vi "模拟发送.vi"() -> ()   [LabVIEW 2013]
panel:
  out "发送成功":bool
  in  "清空":bool
  in  "全选":bool
  in  "DO模块故障":enum16{"无", "一级", "二级", "三级"}(ring) caption="电压检测模块故障"
  in  "DI模块故障":enum16{"无", "一级", "二级", "三级"}(ring) caption="电压检测模块故障"
  in  "软件故障":enum16{"无", "一级", "二级", "三级"}(ring) caption="电压检测模块故障"
  in  "放电均衡模块故障":enum16{"无", "一级", "二级", "三级"}(ring) caption="电压检测模块故障"
  in  "充电均衡模块故障":enum16{"无", "一级", "二级", "三级"}(ring) caption="电压检测模块故障"
  in  "CAN1通讯模块故障":enum16{"无", "一级", "二级", "三级"}(ring) caption="电压检测模块故障"
  in  "CAN0通讯模块故障":enum16{"无", "一级", "二级", "三级"}(ring) caption="电压检测模块故障"
  in  "CAN4通讯模块故障":enum16{"无", "一级", "二级", "三级"}(ring) caption="电压检测模块故障"
  in  "CPU故障":enum16{"无", "一级", "二级", "三级"}(ring) caption="电压检测模块故障"
  in  "CPU内部FLASH存储器故障":enum16{"无", "一级", "二级", "三级"}(ring) caption="电压检测模块故障"
  in  "45db041存储器故障":enum16{"无", "一级", "二级", "三级"}(ring) caption="电压检测模块故障"
  in  "EE存储器故障":enum16{"无", "一级", "二级", "三级"}(ring) caption="电压检测模块故障"
  in  "CPU内部EE故障":enum16{"无", "一级", "二级", "三级"}(ring) caption="电压检测模块故障"
  in  "系统外扩时钟模块故障":enum16{"无", "一级", "二级", "三级"}(ring) caption="电压检测模块故障"
  in  "外总压检测模块故障":enum16{"无", "一级", "二级", "三级"}(ring) caption="电压检测模块故障"
  in  "内总压检测模块故障":enum16{"无", "一级", "二级", "三级"}(ring) caption="电压检测模块故障"
  in  "绝缘检测模块故障":enum16{"无", "一级", "二级", "三级"}(ring) caption="电压检测模块故障"
  in  "电流检测模块故障":enum16{"无", "一级", "二级", "三级"}(ring) caption="电压检测模块故障"
  in  "温度检测模块故障":enum16{"无", "一级", "二级", "三级"}(ring) caption="电压检测模块故障"
  in  "电压检测模块故障":enum16{"无", "一级", "二级", "三级"}(ring)
  in  "默认":bool
  in  "从板板号":T1(ring)
  in  "SOH":i32
  in  "SOC":i32
  in  "放电总安时":dbl
  in  "充电总安时":dbl
  in  "平均电流 2":dbl caption="平均电流"
  in  "外总压 2":dbl caption="外总压"
  in  "总电流 2":dbl caption="总电流"
  in  "总电压 2":dbl caption="总电压"
  out "硬件故障":string
  in  "位置":i32
  in  "最小温度":dbl
  in  "位置":i32
  in  "最大温度":dbl
  in  "位置":i32
  in  "最小电压":dbl
  in  "位置":i32
  in  "最大电压":dbl
  in  "平均电流":dbl
  in  "外总压":dbl
  in  "总电流":dbl
  in  "总电压":dbl
  out "LIFE":i32
  in  "开始":bool
  in  "停止":bool
  # "从板数据"
  # "高压数据"
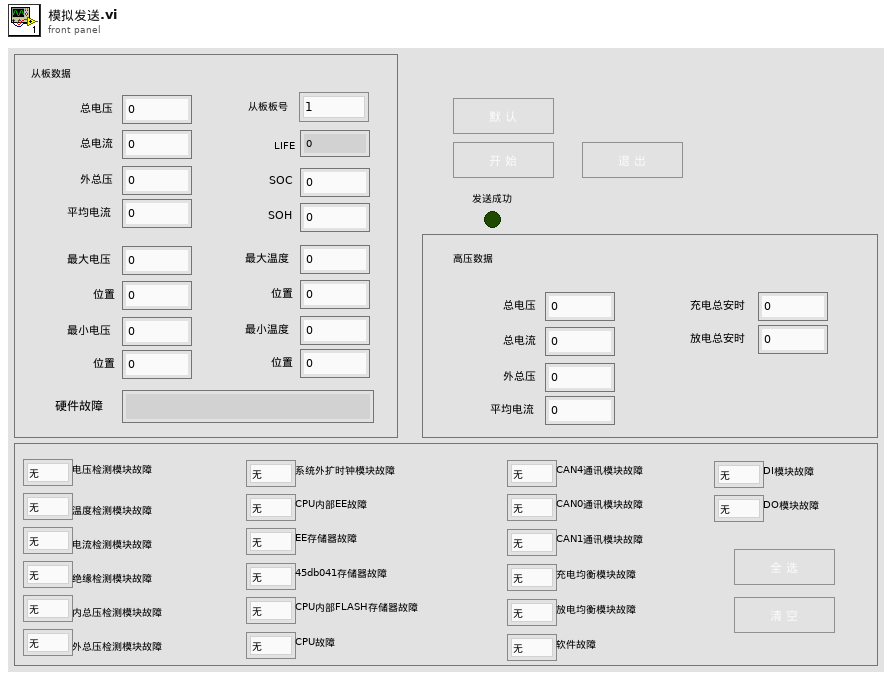
[diagram p1: front panel]
types:
  T1 = enum16{"1", "2", "3", "4", "5", "6", "7", "8", "9", "10", "11", "12", "13", "14", "15", "16", "17", "18", "19", "20", "21", "22", "23", "24", "25", "26", "27", "28", "29", "30"}
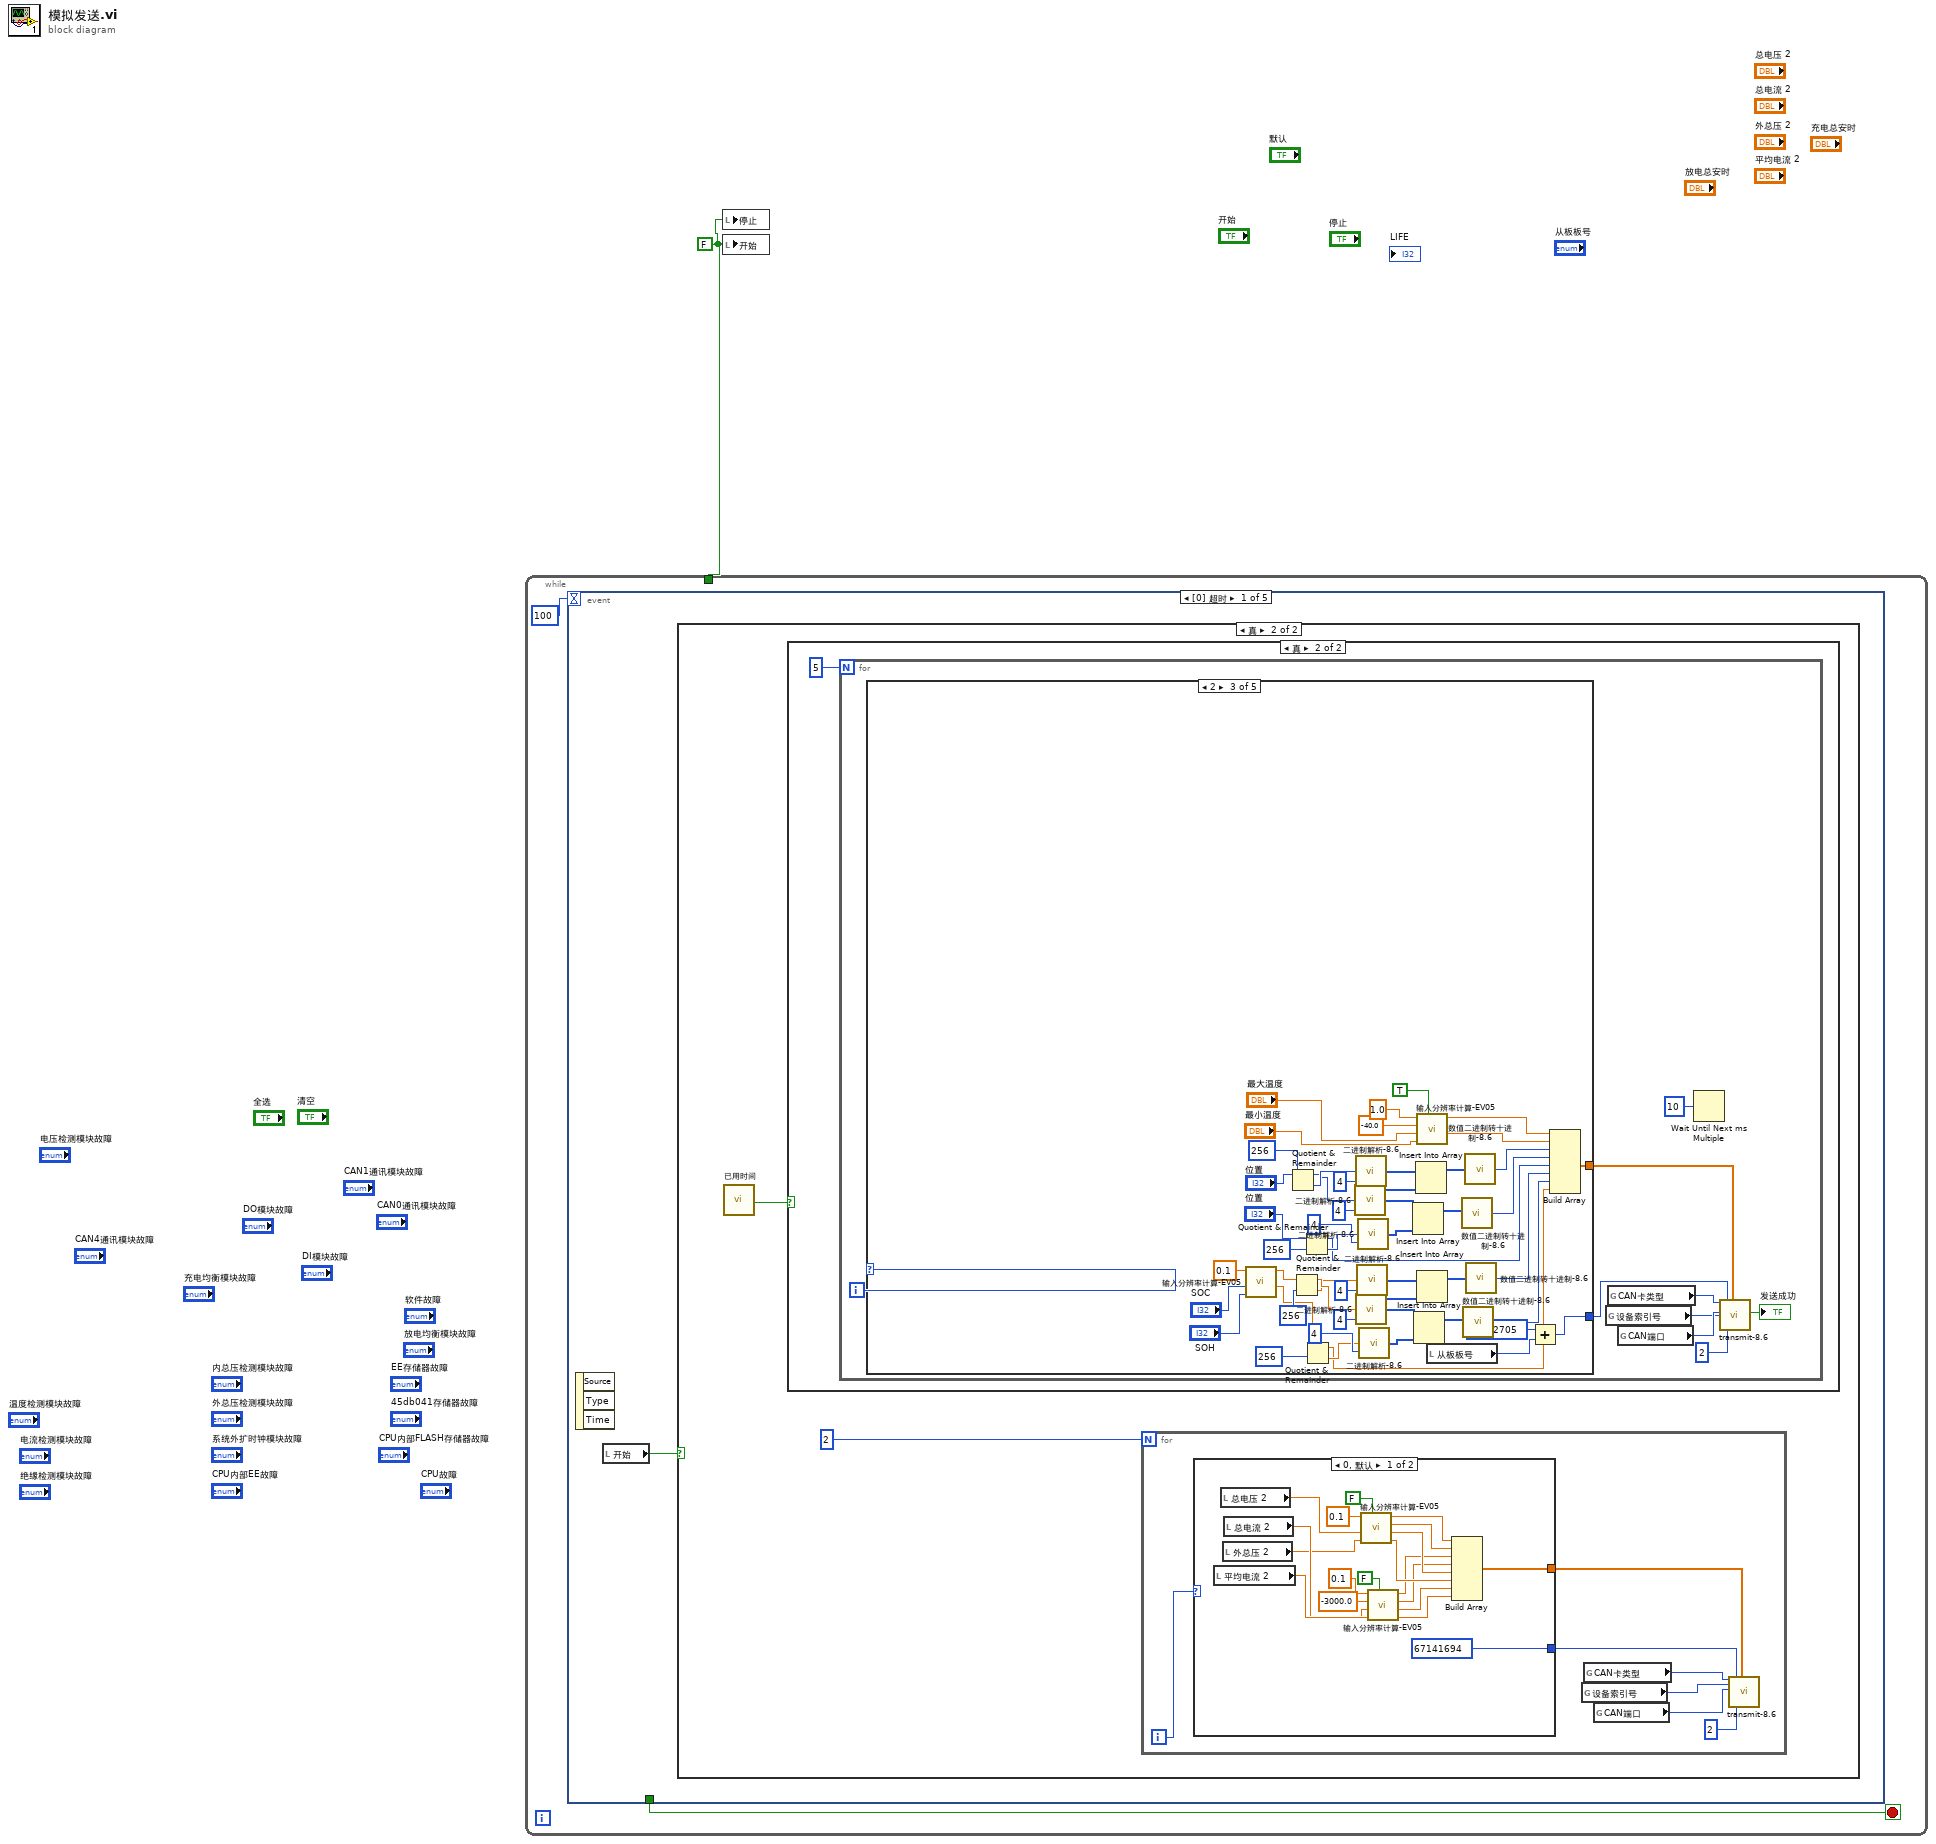
[diagram p0: block diagram]
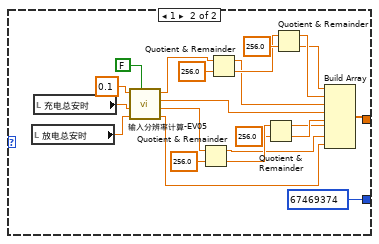
[diagram p3: hidden frame]
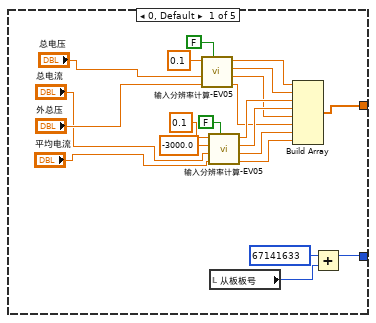
[diagram p5: hidden frame]
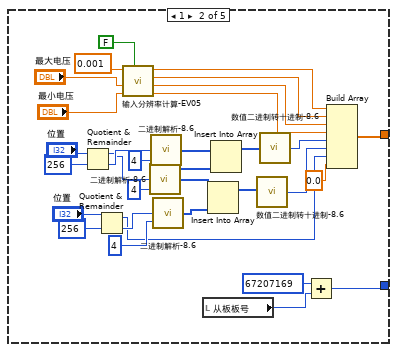
[diagram p6: hidden frame]
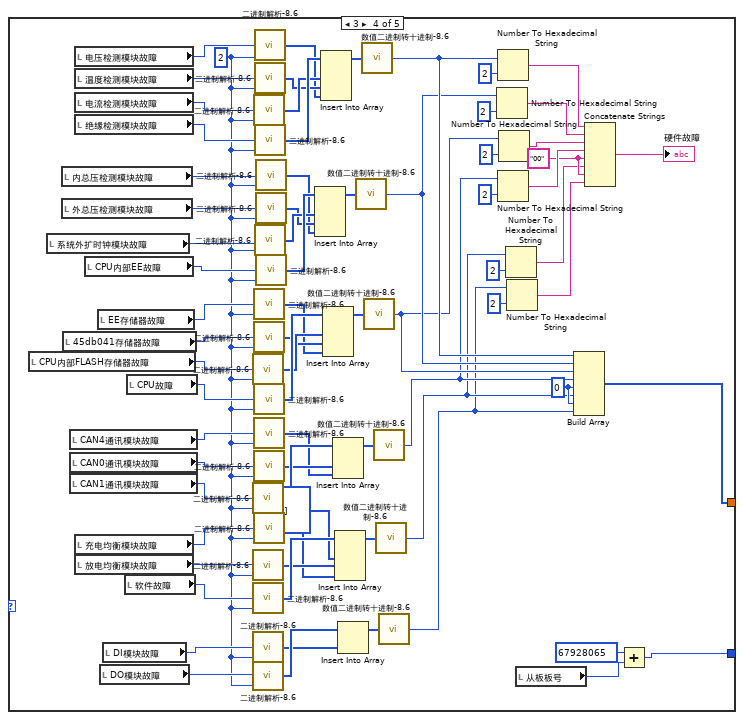
[diagram p7: hidden frame]
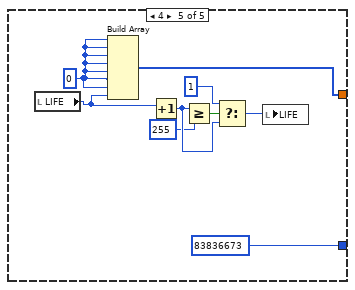
[diagram p8: hidden frame]
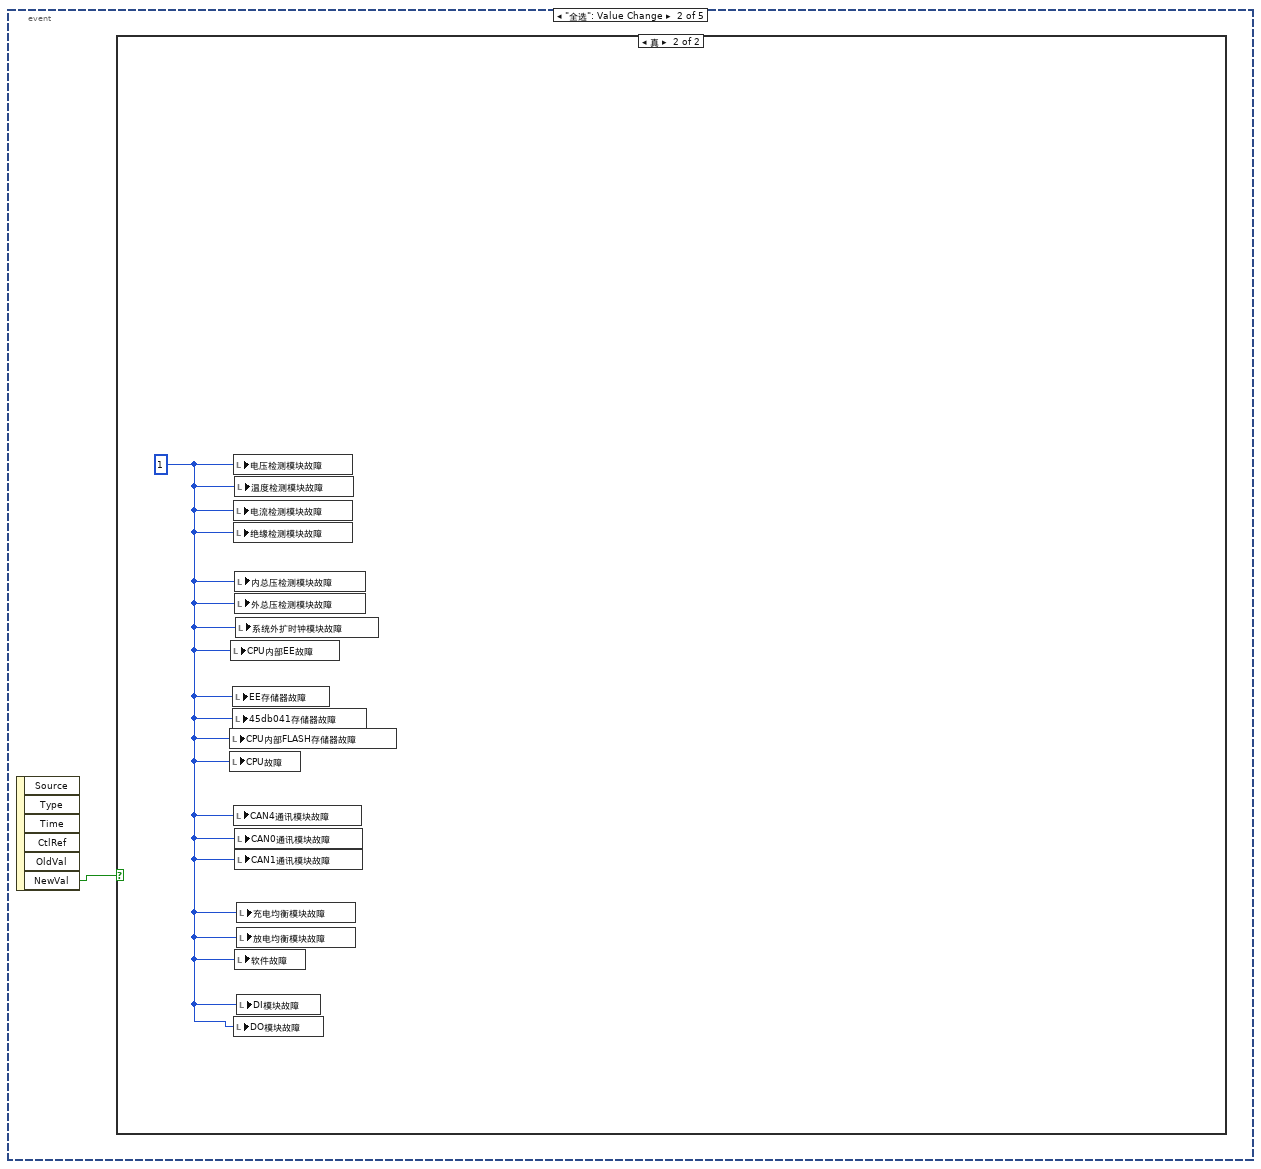
[diagram p9: hidden frame]
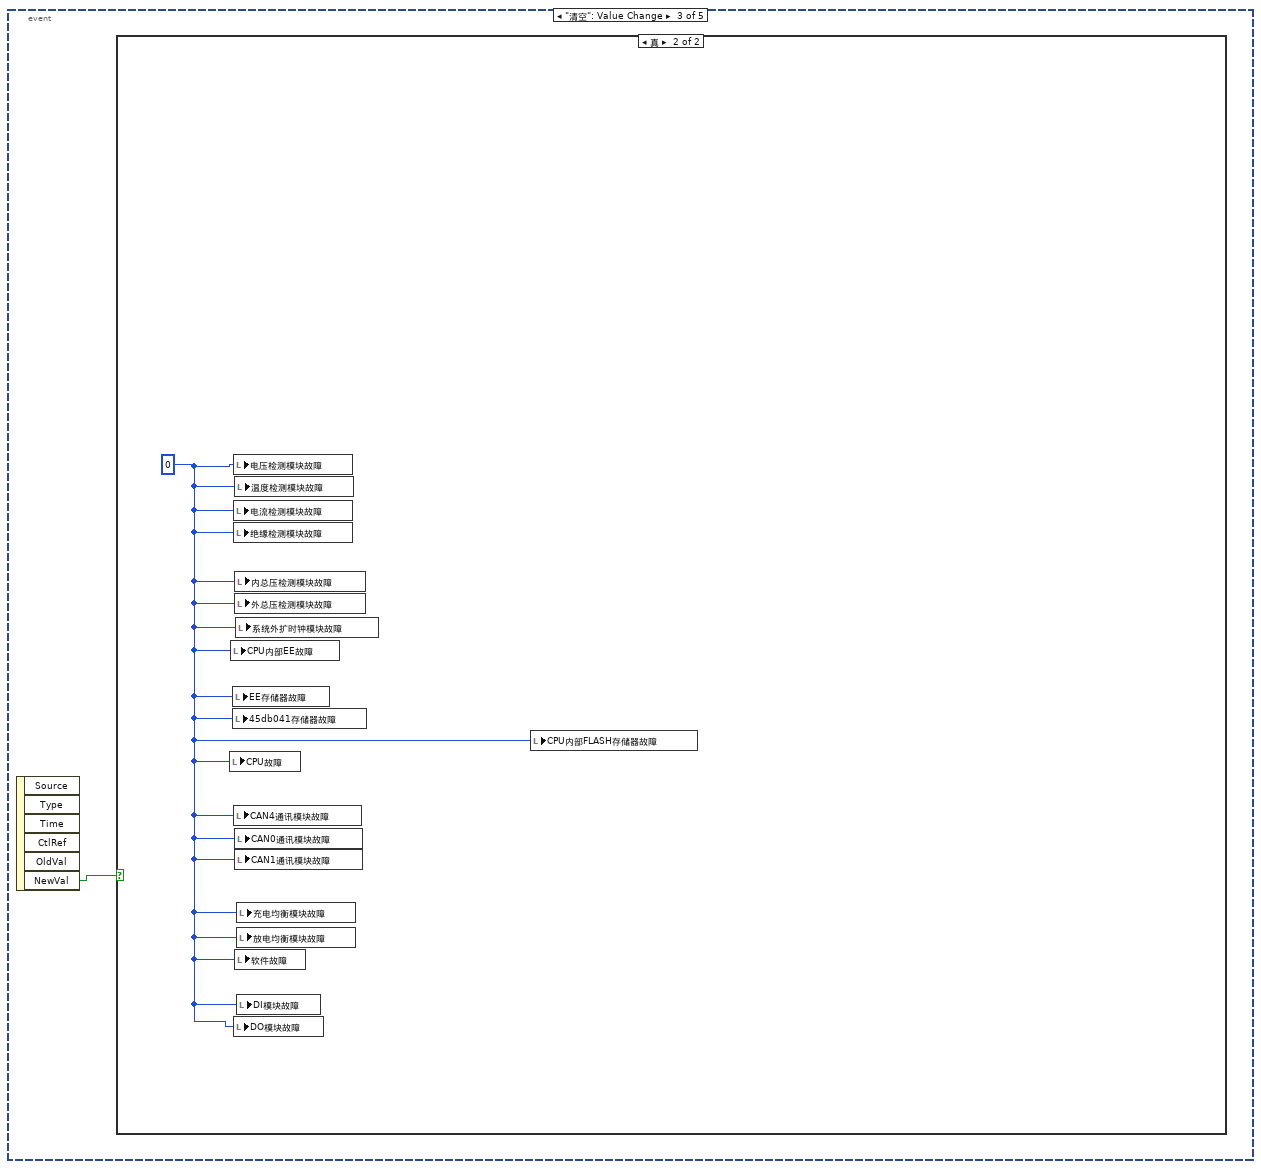
[diagram p11: hidden frame]
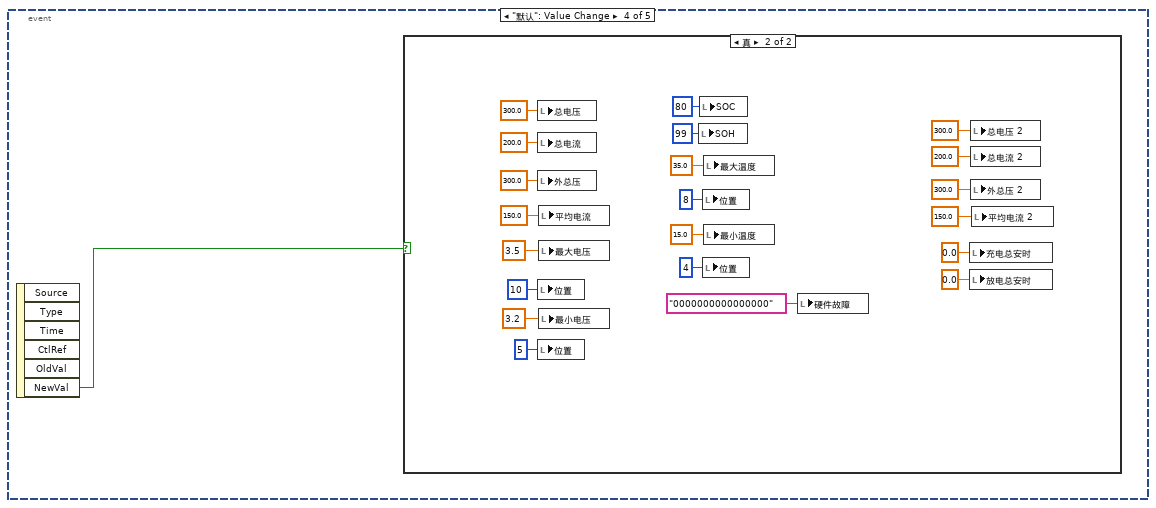
[diagram p13: hidden frame]
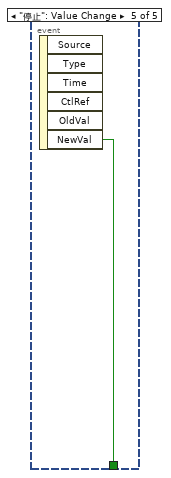
[diagram p15: hidden frame]
diagram:
  w1 = FALSE ("开始")
  n1 = while {
    tunnel: w1 -> [_]
    stop <- w2 stop-if-true
    n2 = event shown="[0] 超时" {
      selector: _ -> [_ _ _ _ _]
      dyn-events: _ -> [_ _ _ _ _]
      timeout: 100 -> [_ _ _ _ _]
      tunnel: [_ _ _ _ w278] -> w2
      event Timeout {
        n3 = event-data() -> ()  [unwired: 1 in, 3 out]
        n4 = local read "开始"() -> (w4:bool)
        n5 = case shown="真" w4 {
          frame False {
          }
          frame True {
            n6 = call "已用时间"() -> ("Time has Elapsed"=w6:bool)  [unwired: 12 in, 7 out]
            n7 = case shown="真" w6 {
              frame False {
              }
              frame True {
                n8 = for {
                  N: 5 -> [_]
                  i -> [w64]
                  n9 = case shown="2" w64 {
                    tunnel: [w69 w113 w169 w190 w244] -> w58
                    tunnel: [w84 w86 w123 w240 83836673] -> w59
                    frame 0, Default {
                      n10 = call "输入分辨率计算-EV05.vi"("1字节?"=FALSE, "数值 2"="外总压", "数值"="总电压", "分辨率"=0.1) -> ("低字节 2"=w72:dbl, "高字节 2"=w73:dbl, "低字节"=w76:dbl, "高字节1"=w77:dbl)  [unwired: 4 in]
                      n11 = call "输入分辨率计算-EV05.vi"("1字节?"=FALSE, "数值 2"="平均电流", "数值"="总电流", "偏移量"=-3000.0, "分辨率"=0.1) -> ("低字节 2"=w70:dbl, "高字节 2"=w71:dbl, "低字节"=w74:dbl, "高字节1"=w75:dbl)  [unwired: 3 in]
                      n12 = local read "从板板号"() -> (w83:T1)
                      n13 = Build Array(w77, w76, w75, w74, w73, w72, w71, w70) -> (w69:dbl[])
                      n14 = Add(x=67141633, y=w83) -> (x+y=w84:i32)
                    }
                    frame 1 {
                      n15 = Quotient & Remainder(x="位置", y=256) -> (x-y*floor(x/y)=w105:i32, floor(x/y)=w108:i32)
                      n16 = Quotient & Remainder(x="位置", y=256) -> (x-y*floor(x/y)=w90:i32, floor(x/y)=w96:i32)
                      n17 = call "输入分辨率计算-EV05.vi"("1字节?"=FALSE, "数值 2"="最小电压", "数值"="最大电压", "分辨率"=0.001) -> ("低字节 2"=w97:dbl, "高字节 2"=w98:dbl, "低字节"=w99:dbl, "高字节1"=w100:dbl)  [unwired: 4 in]
                      n18 = call "二进制解析-8.6.vi"("索引"=4, "数值"=w105) -> ("低位子数组"=w93:i32[], "高位子数组"=w103:i32[])  [unwired: 1 in, 1 out]
                      n19 = call "二进制解析-8.6.vi"("索引"=4, "数值"=w108) -> ("低位子数组"=w104:i32[])  [unwired: 1 in, 2 out]
                      n20 = call "二进制解析-8.6.vi"("索引"=4, "数值"=w96) -> ("低位子数组"=w94:i32[])  [unwired: 1 in, 2 out]
                      n21 = local read "从板板号"() -> (w87:T1)
                      n22 = Insert Into Array(array=w93, new element=w94) -> (w92:i32[])  [unwired: 1 in]
                      n23 = Insert Into Array(array=w104, new element=w103) -> (w102:i32[])  [unwired: 1 in]
                      n24 = call "数值二进制转十进制-8.6.vi"("子数组"=w92) -> ("十进制数值"=w91:i32)  [unwired: 4 in]
                      n25 = call "数值二进制转十进制-8.6.vi"("子数组"=w102) -> ("十进制数值"=w101:i32)  [unwired: 4 in]
                      n26 = Add(x=67207169, y=w87) -> (x+y=w86:i32)
                      n27 = Build Array(w100, w99, w98, w97, w101, w91, w90, 0.0 ("元素")) -> (w113:dbl[])
                    }
                    frame 2 {
                      n28 = call "输入分辨率计算-EV05.vi"("数值 2"="SOH", "数值"="SOC", "分辨率"=0.1) -> ("高字节 2"=w119:dbl, "高字节1"=w120:dbl)  [unwired: 5 in, 2 out]
                      n29 = Quotient & Remainder(x="位置", y=256) -> (x-y*floor(x/y)=w158:i32, floor(x/y)=w161:i32)
                      n30 = Quotient & Remainder(x=w120, y=256) -> (x-y*floor(x/y)=w134:dbl, floor(x/y)=w131:dbl)
                      n31 = Quotient & Remainder(x="位置", y=256) -> (x-y*floor(x/y)=w143:i32, floor(x/y)=w154:i32)
                      n32 = Quotient & Remainder(x=w119, y=256) -> (x-y*floor(x/y)=w128:dbl, floor(x/y)=w138:dbl)
                      n33 = call "二进制解析-8.6.vi"("索引"=4, "数值"=w158) -> ("低位子数组"=w151:i32[], "高位子数组"=w156:i32[])  [unwired: 1 in, 1 out]
                      n34 = call "二进制解析-8.6.vi"("索引"=4, "数值"=w161) -> ("低位子数组"=w157:i32[])  [unwired: 1 in, 2 out]
                      n35 = call "二进制解析-8.6.vi"("索引"=4, "数值"=w134) -> ("低位子数组"=w141:i32[], "高位子数组"=w136:i32[])  [unwired: 1 in, 1 out]
                      n36 = call "二进制解析-8.6.vi"("索引"=4, "数值"=w131) -> ("低位子数组"=w135:i32[])  [unwired: 1 in, 2 out]
                      n37 = call "二进制解析-8.6.vi"("索引"=4, "数值"=w154) -> ("低位子数组"=w152:i32[])  [unwired: 1 in, 2 out]
                      n38 = call "二进制解析-8.6.vi"("索引"=4, "数值"=w138) -> ("低位子数组"=w140:i32[])  [unwired: 1 in, 2 out]
                      n39 = Insert Into Array(array=w151, new element=w152) -> (w150:i32[])  [unwired: 1 in]
                      n40 = Insert Into Array(array=w141, new element=w140) -> (w142:i32[])  [unwired: 1 in]
                      n41 = Insert Into Array(array=w157, new element=w156) -> (w155:i32[])  [unwired: 1 in]
                      n42 = call "输入分辨率计算-EV05.vi"("1字节?"=TRUE, "数值 2"="最小温度", "数值"="最大温度", "偏移量"=-40.0, "分辨率"=1.0) -> ("高字节 2"=w162:dbl, "高字节1"=w163:dbl)  [unwired: 3 in, 2 out]
                      n43 = Insert Into Array(array=w135, new element=w136) -> (w137:i32[])  [unwired: 1 in]
                      n44 = local read "从板板号"() -> (w124:T1)
                      n45 = call "数值二进制转十进制-8.6.vi"("子数组"=w150) -> ("十进制数值"=w144:i32)  [unwired: 4 in]
                      n46 = call "数值二进制转十进制-8.6.vi"("子数组"=w142) -> ("十进制数值"=w127:i32)  [unwired: 4 in]
                      n47 = call "数值二进制转十进制-8.6.vi"("子数组"=w155) -> ("十进制数值"=w145:i32)  [unwired: 4 in]
                      n48 = call "数值二进制转十进制-8.6.vi"("子数组"=w137) -> ("十进制数值"=w126:i32)  [unwired: 4 in]
                      n49 = Add(x=67272705, y=w124) -> (x+y=w123:i32)
                      n50 = Build Array(w163, w162, w145, w144, w143, w126, w127, w128) -> (w169:dbl[])
                    }
                    frame 3 {
                      w172 = "00" ("字符串")
                      w189 = 0 ("元素")
                      w219 = 2
                      n51 = local read "CPU内部FLASH存储器故障"() -> (w229:enum16{"无", "一级", "二级", "三级"})
                      n52 = local read "系统外扩时钟模块故障"() -> (w233:enum16{"无", "一级", "二级", "三级"})
                      n53 = local read "内总压检测模块故障"() -> (w235:enum16{"无", "一级", "二级", "三级"})
                      n54 = local read "外总压检测模块故障"() -> (w234:enum16{"无", "一级", "二级", "三级"})
                      n55 = local read "45db041存储器故障"() -> (w230:enum16{"无", "一级", "二级", "三级"})
                      n56 = local read "CAN4通讯模块故障"() -> (w227:enum16{"无", "一级", "二级", "三级"})
                      n57 = local read "CAN0通讯模块故障"() -> (w226:enum16{"无", "一级", "二级", "三级"})
                      n58 = local read "CAN1通讯模块故障"() -> (w225:enum16{"无", "一级", "二级", "三级"})
                      n59 = local read "电压检测模块故障"() -> (w239:enum16{"无", "一级", "二级", "三级"})
                      n60 = local read "温度检测模块故障"() -> (w238:enum16{"无", "一级", "二级", "三级"})
                      n61 = local read "电流检测模块故障"() -> (w237:enum16{"无", "一级", "二级", "三级"})
                      n62 = local read "绝缘检测模块故障"() -> (w236:enum16{"无", "一级", "二级", "三级"})
                      n63 = local read "充电均衡模块故障"() -> (w224:enum16{"无", "一级", "二级", "三级"})
                      n64 = local read "放电均衡模块故障"() -> (w223:enum16{"无", "一级", "二级", "三级"})
                      n65 = local read "CPU内部EE故障"() -> (w232:enum16{"无", "一级", "二级", "三级"})
                      n66 = local read "EE存储器故障"() -> (w231:enum16{"无", "一级", "二级", "三级"})
                      n67 = local read "DO模块故障"() -> (w220:enum16{"无", "一级", "二级", "三级"})
                      n68 = local read "DI模块故障"() -> (w221:enum16{"无", "一级", "二级", "三级"})
                      n69 = local read "软件故障"() -> (w222:enum16{"无", "一级", "二级", "三级"})
                      n70 = local read "CPU故障"() -> (w228:enum16{"无", "一级", "二级", "三级"})
                      n71 = call "二进制解析-8.6.vi"("索引"=w219, "数值"=w229) -> ("低位子数组"=w202:i32[])  [unwired: 1 in, 2 out]
                      n72 = call "二进制解析-8.6.vi"("索引"=w219, "数值"=w225) -> ("低位子数组"=w198:i32[])  [unwired: 1 in, 2 out]
                      n73 = call "二进制解析-8.6.vi"("索引"=w219, "数值"=w223) -> ("低位子数组"=w193:i32[])  [unwired: 1 in, 2 out]
                      n74 = call "二进制解析-8.6.vi"("索引"=w219, "数值"=w222) -> ("低位子数组"=w194:i32[])  [unwired: 1 in, 2 out]
                      n75 = call "二进制解析-8.6.vi"("索引"=w219, "数值"=w221) -> ("低位子数组"=w186:i32[])  [unwired: 1 in, 2 out]
                      n76 = call "二进制解析-8.6.vi"("索引"=w219, "数值"=w220) -> ("低位子数组"=w187:i32[])  [unwired: 1 in, 2 out]
                      n77 = call "二进制解析-8.6.vi"("索引"=w219, "数值"=w237) -> ("低位子数组"=w211:i32[])  [unwired: 1 in, 2 out]
                      n78 = call "二进制解析-8.6.vi"("索引"=w219, "数值"=w231) -> ("低位子数组"=w200:i32[])  [unwired: 1 in, 2 out]
                      n79 = call "二进制解析-8.6.vi"("索引"=w219, "数值"=w230) -> ("低位子数组"=w201:i32[])  [unwired: 1 in, 2 out]
                      n80 = call "二进制解析-8.6.vi"("索引"=w219, "数值"=w228) -> ("低位子数组"=w203:i32[])  [unwired: 1 in, 2 out]
                      n81 = call "二进制解析-8.6.vi"("索引"=w219, "数值"=w227) -> ("低位子数组"=w196:i32[])  [unwired: 1 in, 2 out]
                      n82 = call "二进制解析-8.6.vi"("索引"=w219, "数值"=w226) -> ("低位子数组"=w197:i32[])  [unwired: 1 in, 2 out]
                      n83 = call "二进制解析-8.6.vi"("索引"=w219, "数值"=w224) -> ("低位子数组"=w192:i32[])  [unwired: 1 in, 2 out]
                      n84 = call "二进制解析-8.6.vi"("索引"=w219, "数值"=w239) -> ("低位子数组"=w209:i32[])  [unwired: 1 in, 2 out]
                      n85 = call "二进制解析-8.6.vi"("索引"=w219, "数值"=w238) -> ("低位子数组"=w210:i32[])  [unwired: 1 in, 2 out]
                      n86 = call "二进制解析-8.6.vi"("索引"=w219, "数值"=w236) -> ("低位子数组"=w212:i32[])  [unwired: 1 in, 2 out]
                      n87 = call "二进制解析-8.6.vi"("索引"=w219, "数值"=w233) -> ("低位子数组"=w207:i32[])  [unwired: 1 in, 2 out]
                      n88 = call "二进制解析-8.6.vi"("索引"=w219, "数值"=w235) -> ("低位子数组"=w205:i32[])  [unwired: 1 in, 2 out]
                      n89 = call "二进制解析-8.6.vi"("索引"=w219, "数值"=w234) -> ("低位子数组"=w206:i32[])  [unwired: 1 in, 2 out]
                      n90 = call "二进制解析-8.6.vi"("索引"=w219, "数值"=w232) -> ("低位子数组"=w208:i32[])  [unwired: 1 in, 2 out]
                      n91 = Insert Into Array(array=w208, new element #1=w207, new element #2=w206, new element #3=w205) -> (w213:i32[])  [unwired: 1 in]
                      n92 = Insert Into Array(array=w212, new element #1=w211, new element #2=w210, new element #3=w209) -> (w218:i32[])  [unwired: 1 in]
                      n93 = Insert Into Array(array=w203, new element #1=w202, new element #2=w201, new element #3=w200) -> (w204:i32[])  [unwired: 1 in]
                      n94 = Insert Into Array(array=w198, new element #1=w197, new element #2=w196) -> (w199:i32[])  [unwired: 1 in]
                      n95 = Insert Into Array(array=w194, new element #1=i32[] [0, 0], new element #2=w193, new element #3=w192) -> (w195:i32[])  [unwired: 1 in]
                      n96 = Insert Into Array(array=w187, new element=w186) -> (w188:i32[])  [unwired: 1 in]
                      n97 = call "数值二进制转十进制-8.6.vi"("子数组"=w213) -> ("十进制数值"=w180:i32)  [unwired: 4 in]
                      n98 = call "数值二进制转十进制-8.6.vi"("子数组"=w218) -> ("十进制数值"=w214:i32)  [unwired: 4 in]
                      n99 = call "数值二进制转十进制-8.6.vi"("子数组"=w204) -> ("十进制数值"=w179:i32)  [unwired: 4 in]
                      n100 = call "数值二进制转十进制-8.6.vi"("子数组"=w199) -> ("十进制数值"=w178:i32)  [unwired: 4 in]
                      n101 = call "数值二进制转十进制-8.6.vi"("子数组"=w195) -> ("十进制数值"=w177:i32)  [unwired: 4 in]
                      n102 = call "数值二进制转十进制-8.6.vi"("子数组"=w188) -> ("十进制数值"=w176:i32)  [unwired: 4 in]
                      n103 = Number To Hexadecimal String(1:i16 2 ("宽度(-)"), 2:w180) -> (0:w175:string)
                      n104 = Number To Hexadecimal String(1:i16 2 ("宽度(-)"), 2:w214) -> (0:w216:string)
                      n105 = Number To Hexadecimal String(1:i16 2 ("宽度(-)"), 2:w178) -> (0:w173:string)
                      n106 = Number To Hexadecimal String(1:i16 2 ("宽度(-)"), 2:w179) -> (0:w174:string)
                      n107 = Number To Hexadecimal String(1:i16 2 ("宽度(-)"), 2:w177) -> (0:w171:string)
                      n108 = Number To Hexadecimal String(1:i16 2 ("宽度(-)"), 2:w176) -> (0:w170:string)
                      n109 = local read "从板板号"() -> (w241:T1)
                      n110 = Build Array(w214, w180, w179, w178, w189, w177, w189, w176) -> (w190:i32[])
                      n111 = Concatenate Strings(w216, w175, w174, w173, w172, w171, w172, w170) -> (→"硬件故障":string)
                      n112 = Add(x=67928065, y=w241) -> (x+y=w240:i32)
                    }
                    frame 4 {
                      w245 = 0
                      n113 = local read "LIFE"() -> (w246:i32)
                      n114 = Build Array(w245, w245, w245, w245, w245, w245, w245, w246) -> (w244:i32[])
                      n115 = Increment(x=w246) -> (x+1=w251:i32)
                      n116 = Greater Or Equal?(x=w251, y=255) -> (x >= y?=w248:bool)
                      n117 = Select(t=1 ("y"), s=w248, f=w251) -> (s? t:f=w250:i32)
                      n118 = local write "LIFE"(w250) -> ()
                    }
                  }
                  n119 = global read "EV05全局变量1.vi" "设备索引号"() -> (w61:u16)
                  n120 = global read "EV05全局变量1.vi" "CAN卡类型"() -> (w60:u32)
                  n121 = global read "EV05全局变量1.vi" "CAN端口"() -> (w62:u16)
                  n122 = Wait Until Next ms Multiple(millisecond multiple=u32 10 ("毫秒倍数")) -> ()  [unwired: 1 out]
                  n123 = call "transmit-8.6.vi"("can卡类型"=w60, "设备索引号"=w61, "CAN端口"=w62, "ID"=w59, "SendType"=u8 2, "Data"=w58) -> ("发送成功"=→"发送成功":bool)  [unwired: 3 in, 10 out]
                }
              }
            }
            n124 = for {
              N: 2 -> [_]
              i -> [w13]
              n125 = case shown="0, 默认" w13 {
                tunnel: [w15 w50] -> w8
                tunnel: [67141694 67469374] -> w7
                frame 0, Default {
                  n126 = local read "平均电流 2"() -> (w19:dbl)
                  n127 = local read "总电压 2"() -> (w16:dbl)
                  n128 = local read "外总压 2"() -> (w17:dbl)
                  n129 = local read "总电流 2"() -> (w18:dbl)
                  n130 = call "输入分辨率计算-EV05.vi"("1字节?"=FALSE, "数值 2"=w17, "数值"=w16, "分辨率"=0.1) -> ("低字节 2"=w30:dbl, "高字节 2"=w29:dbl, "低字节"=w26:dbl, "高字节1"=w25:dbl)  [unwired: 4 in]
                  n131 = call "输入分辨率计算-EV05.vi"("1字节?"=FALSE, "数值 2"=w19, "数值"=w18, "偏移量"=-3000.0, "分辨率"=0.1) -> ("低字节 2"=w32:dbl, "高字节 2"=w31:dbl, "低字节"=w28:dbl, "高字节1"=w27:dbl)  [unwired: 3 in]
                  n132 = Build Array(w25, w26, w27, w28, w29, w30, w31, w32) -> (w15:dbl[])
                }
                frame 1 {
                  n133 = local read "放电总安时"() -> (w53:dbl)
                  n134 = local read "充电总安时"() -> (w54:dbl)
                  n135 = call "输入分辨率计算-EV05.vi"("1字节?"=FALSE, "数值 2"=w53, "数值"=w54, "分辨率"=0.1) -> ("低字节 2"=w36:dbl, "高字节 2"=w37:dbl, "低字节"=w44:dbl, "高字节1"=w47:dbl)  [unwired: 4 in]
                  n136 = Quotient & Remainder(x=w37, y=256.0) -> (x-y*floor(x/y)=w35:dbl, floor(x/y)=w40:dbl)
                  n137 = Quotient & Remainder(x=w47, y=256.0) -> (x-y*floor(x/y)=w43:dbl, floor(x/y)=w45:dbl)
                  n138 = Quotient & Remainder(x=w40, y=256.0) -> (x-y*floor(x/y)=w33:dbl, floor(x/y)=w34:dbl)
                  n139 = Quotient & Remainder(x=w45, y=256.0) -> (x-y*floor(x/y)=w42:dbl, floor(x/y)=w41:dbl)
                  n140 = Build Array(w41, w42, w43, w44, w34, w33, w35, w36) -> (w50:dbl[])
                }
              }
              n141 = global read "EV05全局变量1.vi" "设备索引号"() -> (w11:u16)
              n142 = global read "EV05全局变量1.vi" "CAN卡类型"() -> (w12:u32)
              n143 = global read "EV05全局变量1.vi" "CAN端口"() -> (w10:u16)
              n144 = call "transmit-8.6.vi"("can卡类型"=w12, "设备索引号"=w11, "CAN端口"=w10, "ID"=w7, "SendType"=u8 2, "Data"=w8) -> ()  [unwired: 3 in, 11 out]
            }
          }
        }
      }
      event "全选": Value Change {
        n145 = event-data() -> ("NewVal"=w252:bool)  [unwired: 1 in, 5 out]
        n146 = case shown="真" w252 {
          frame False {
          }
          frame True {
            w253 = 1
            n147 = local write "CPU内部FLASH存储器故障"(w253) -> ()
            n148 = local write "CPU故障"(w253) -> ()
            n149 = local write "CPU内部EE故障"(w253) -> ()
            n150 = local write "EE存储器故障"(w253) -> ()
            n151 = local write "45db041存储器故障"(w253) -> ()
            n152 = local write "电压检测模块故障"(w253) -> ()
            n153 = local write "电流检测模块故障"(w253) -> ()
            n154 = local write "绝缘检测模块故障"(w253) -> ()
            n155 = local write "CAN4通讯模块故障"(w253) -> ()
            n156 = local write "DO模块故障"(w253) -> ()
            n157 = local write "温度检测模块故障"(w253) -> ()
            n158 = local write "内总压检测模块故障"(w253) -> ()
            n159 = local write "外总压检测模块故障"(w253) -> ()
            n160 = local write "CAN0通讯模块故障"(w253) -> ()
            n161 = local write "CAN1通讯模块故障"(w253) -> ()
            n162 = local write "软件故障"(w253) -> ()
            n163 = local write "系统外扩时钟模块故障"(w253) -> ()
            n164 = local write "充电均衡模块故障"(w253) -> ()
            n165 = local write "放电均衡模块故障"(w253) -> ()
            n166 = local write "DI模块故障"(w253) -> ()
          }
        }
      }
      event "清空": Value Change {
        n167 = event-data() -> ("NewVal"=w254:bool)  [unwired: 1 in, 5 out]
        n168 = case shown="真" w254 {
          frame False {
          }
          frame True {
            w255 = 0
            n169 = local write "CPU故障"(w255) -> ()
            n170 = local write "CPU内部EE故障"(w255) -> ()
            n171 = local write "EE存储器故障"(w255) -> ()
            n172 = local write "45db041存储器故障"(w255) -> ()
            n173 = local write "电压检测模块故障"(w255) -> ()
            n174 = local write "电流检测模块故障"(w255) -> ()
            n175 = local write "绝缘检测模块故障"(w255) -> ()
            n176 = local write "CAN4通讯模块故障"(w255) -> ()
            n177 = local write "DO模块故障"(w255) -> ()
            n178 = local write "温度检测模块故障"(w255) -> ()
            n179 = local write "内总压检测模块故障"(w255) -> ()
            n180 = local write "外总压检测模块故障"(w255) -> ()
            n181 = local write "CAN0通讯模块故障"(w255) -> ()
            n182 = local write "CAN1通讯模块故障"(w255) -> ()
            n183 = local write "软件故障"(w255) -> ()
            n184 = local write "系统外扩时钟模块故障"(w255) -> ()
            n185 = local write "充电均衡模块故障"(w255) -> ()
            n186 = local write "放电均衡模块故障"(w255) -> ()
            n187 = local write "DI模块故障"(w255) -> ()
            n188 = local write "CPU内部FLASH存储器故障"(w255) -> ()
          }
        }
      }
      event "默认": Value Change {
        n189 = event-data() -> ("NewVal"=w256:bool)  [unwired: 1 in, 5 out]
        n190 = case shown="真" w256 {
          frame False {
          }
          frame True {
            n191 = local write "总电压"(300.0 ("总电压")) -> ()
            n192 = local write "总电流"(200.0 ("总电流")) -> ()
            n193 = local write "外总压"(300.0 ("外总压")) -> ()
            n194 = local write "位置"(10 ("位置")) -> ()
            n195 = local write "位置"(5 ("位置")) -> ()
            n196 = local write "平均电流"(150.0 ("平均电流")) -> ()
            n197 = local write "最大电压"(3.5 ("最大电压")) -> ()
            n198 = local write "最小电压"(3.2 ("最小电压")) -> ()
            n199 = local write "SOH"(99 ("SOH")) -> ()
            n200 = local write "SOC"(80 ("SOC")) -> ()
            n201 = local write "位置"(8 ("位置")) -> ()
            n202 = local write "位置"(4 ("位置")) -> ()
            n203 = local write "最大温度"(35.0 ("最大温度")) -> ()
            n204 = local write "最小温度"(15.0 ("最小温度")) -> ()
            n205 = local write "硬件故障"("0000000000000000" ("硬件故障")) -> ()
            n206 = local write "充电总安时"(0.0 ("充电总安时")) -> ()
            n207 = local write "放电总安时"(0.0 ("放电总安时")) -> ()
            n208 = local write "总电压 2"(300.0 ("总电压 2")) -> ()
            n209 = local write "总电流 2"(200.0 ("总电流 2")) -> ()
            n210 = local write "外总压 2"(300.0 ("外总压 2")) -> ()
            n211 = local write "平均电流 2"(150.0 ("平均电流 2")) -> ()
          }
        }
      }
      event "停止": Value Change {
        n212 = event-data() -> ("NewVal"=w278:bool)  [unwired: 1 in, 5 out]
      }
    }
  }
  n213 = local write "停止"(w1) -> ()
  n214 = local write "开始"(w1) -> ()
